vi "FGV.vi"(6 "Variant":variant, 7 "Connection Information":string, 8 "error in (no error)":errorcluster, 9 "column information":T1[](array[typedef])=[{"column name"="", "data type"=enum."Double (DBL)", "size"=0, "allow null?"=TRUE}], 10 "table":string, 11 "Enum":T3(ring)) -> (0 "error out":errorcluster, 1 "data":string[][](array[string]), 3 "tables":string[](array[string]))   [LabVIEW 2014]
uses:
  <vilib>/addons/database/NI_Database_API.lvlib
  <vilib>/addons/database/Connection.llb/Conn ObjectReference.ctl
  <vilib>/addons/database/_DB Variant To Data/Database Variant To Data.xnode
  SEQ/SeqLoop/TypeDefs/HW InOut MAP.ctl
  SEQ/SeqLoop/SeqLoop.lvlib
  SEQ/SeqLoop/Classes/STEP/STEP.lvclass
  SEQ/SeqLoop/TypeDefs/LogicParsedExpression.ctl
  SEQ/SeqLoop/TypeDefs/Sequence.ctl
  SEQ/SeqLoop/TypeDefs/Program.ctl
  <vilib>/addons/database/Connection.llb/Conn Transaction.vi
  <vilib>/addons/database/Auxilliary.llb/DB Tools Transaction.ctl
  <vilib>/addons/database/Connection.llb/DB Tools Open Connec (String).vi
  <vilib>/addons/database/Auxilliary.llb/DB Tools DataTypes.ctl
  <vilib>/addons/database/Auxilliary.llb/DB Tools Column Info.ctl
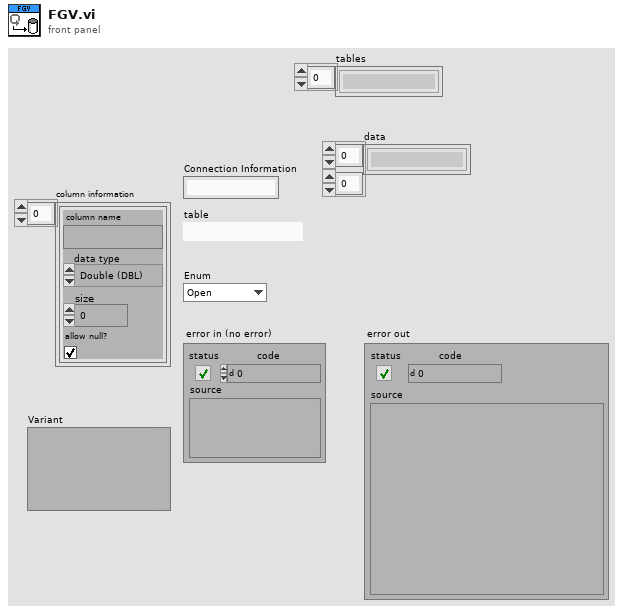
[diagram p1: front panel]
types:
  T1 = typedef "NI_Database_API.lvlib/DB Tools Column Info.ctl" = cluster{"column name":string, "data type":T2, "size":i32, "allow null?":bool}
  T2 = typedef "NI_Database_API.lvlib/DB Tools DataTypes.ctl" = enum16{"String", "Long (I32)", "Single (SGL)", "Double (DBL)", "Date/Time", "Binary"}
  T3 = enum16{"Open", "Create", "Delete", "Read_HAL", "Read_CORE", "Read_UI", "Read_MATH", "Read_SEQ", "Write_HAL", "Write_CORE", "Write_UI", "Write_MATH", "Write_SEQ", "Close"}
  T4 = typedef "NI_Database_API.lvlib/DB Tools Transaction.ctl" = enum16{"begin", "commit", "rollback"}
  T5 = typedef "NI_Database_API.lvlib/Conn ObjectReference.ctl" = refnum<k1>
  T6 = typedef "SeqLoop.lvlib/Program.ctl" = cluster{"Prog. Data":cluster{"Tipo de Programa":string, "Operación":i32, "Pieza":i32, "Descripción":string, "Nombre Programa":string, "Autor":string, "Cód. Prog.":i32, "Diseño":string, "Total Meds.:":i32, "Total Meds. Aux.:":i32}, "All Sequences":cluster{"Measurement":T7, "AutoZero":T7, "Special":T7}}
  T7 = typedef "SeqLoop.lvlib/Sequence.ctl" = cluster{"STEPs":refnum<class "STEP.lvclass">[], "Main Error&Alarm":cluster{"Main Error":T8, "Main Alarm 1":T8, "Main Alarm 2":T8, "Main Alarm 3":T8, "Main Alarm 4":T8}, "STEP Type":refnum<class "STEP.lvclass">}
  T8 = typedef "SeqLoop.lvlib/LogicParsedExpression.ctl" = cluster{"RPN ":string[], "Variables":string[], "Ctes":string[], "Formula":string, "Message":string}
  T9 = typedef "SeqLoop.lvlib/HW InOut MAP.ctl" = cluster{"Inputs":cluster{"Entrada":i32, "Descripción":string, "Habilitada?":bool}[][], "Outputs":cluster{"Salida":i32, "Descripción":string, "Habilitada?":bool, "Formula":string, "Tipo de Salida":string}[][]}
  T10 = cluster{"Entrada":i32, "Descripción":string, "Habilitada?":bool}[][]
  T11 = cluster{string, string, string, "Descripción":string, "Descripción":string}
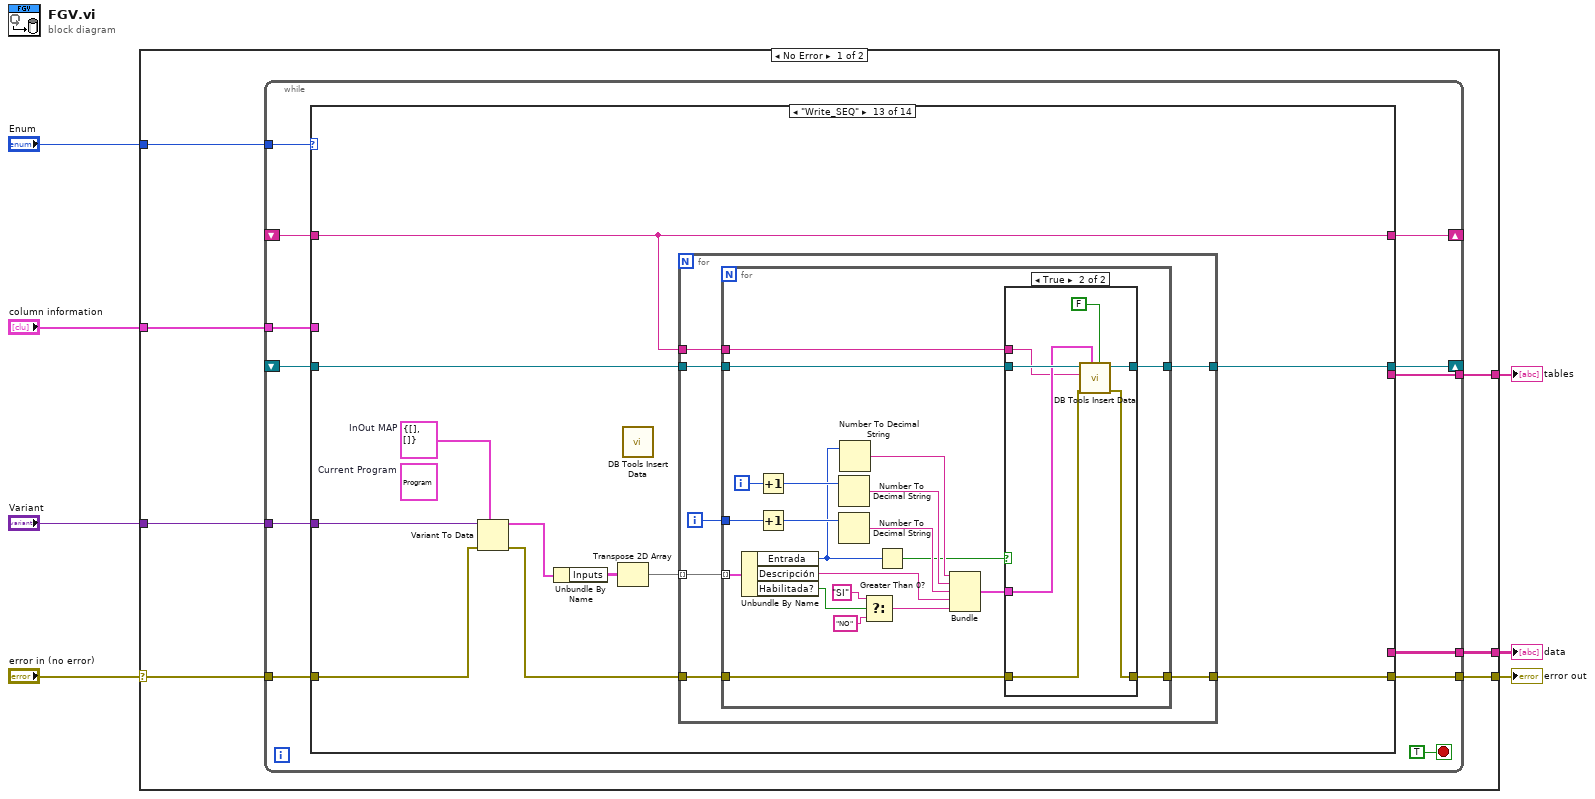
[diagram p0: block diagram]
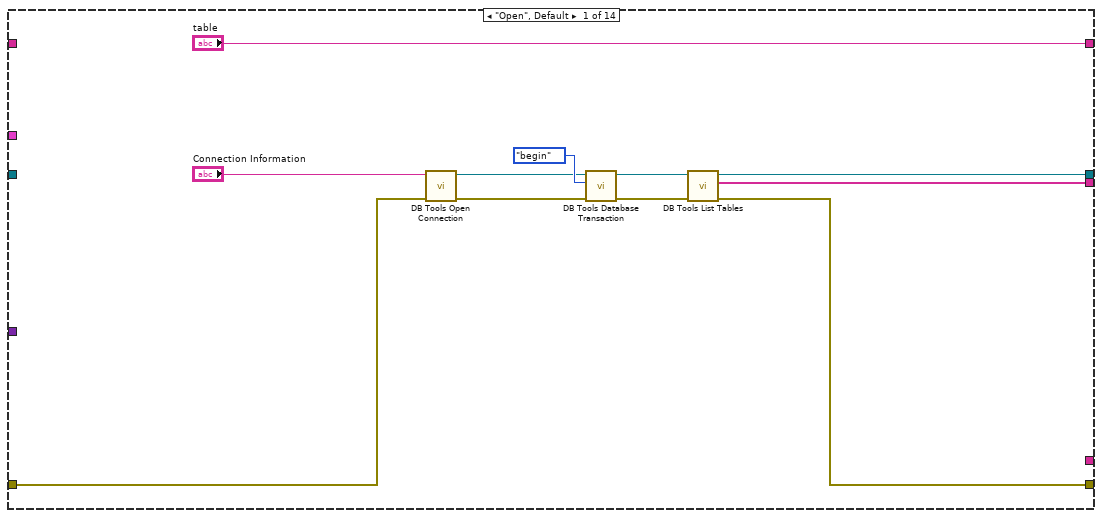
[diagram p2: hidden frame]
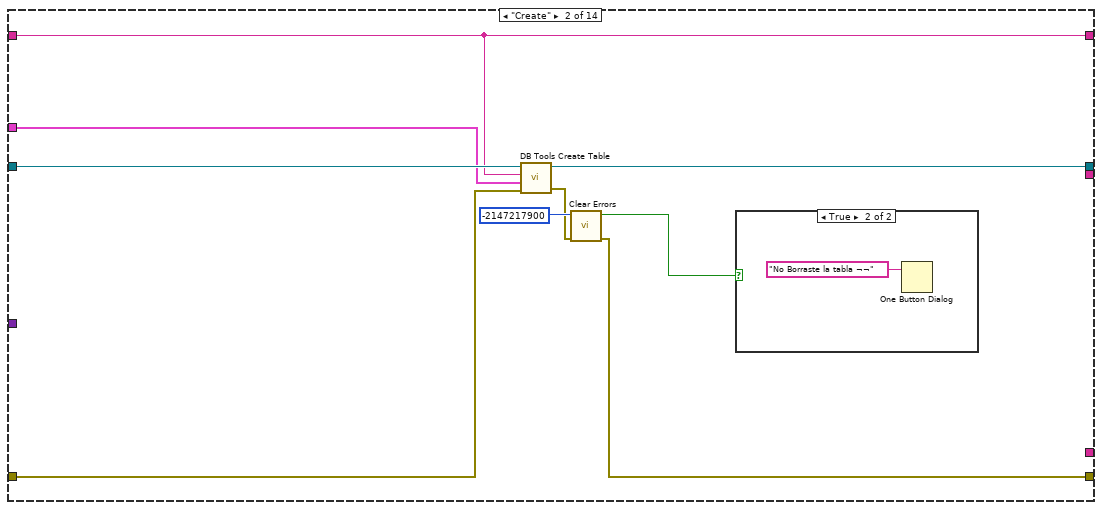
[diagram p3: hidden frame]
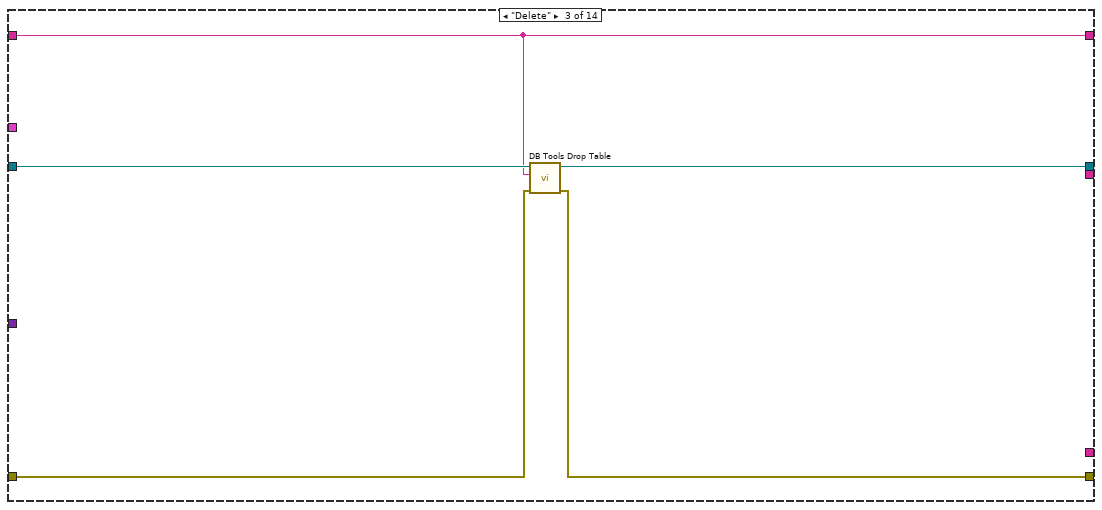
[diagram p5: hidden frame]
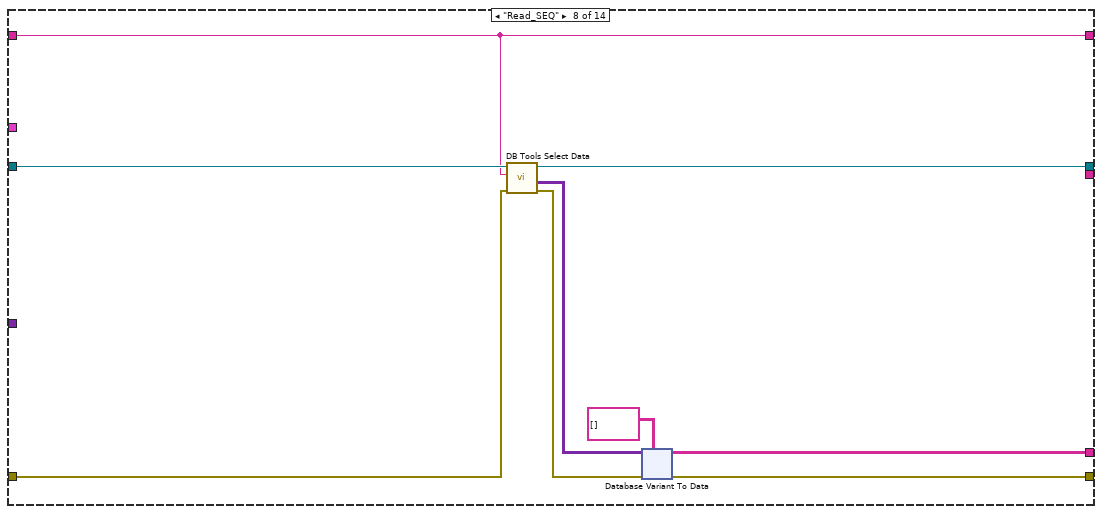
[diagram p10: hidden frame]
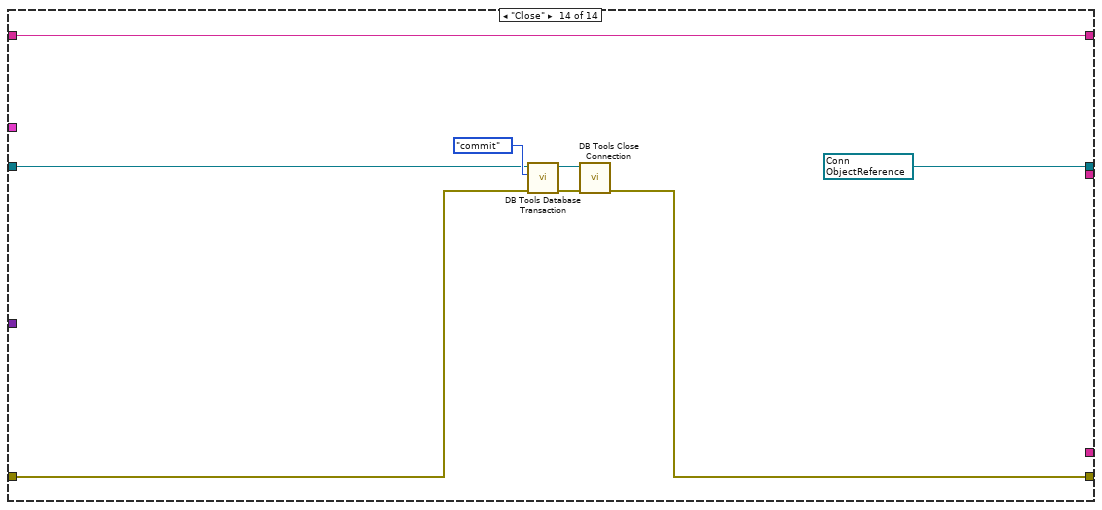
[diagram p16: hidden frame]
diagram:
  n1 = case shown="No Error" "error in (no error)" {
    selector: "error in (no error)" -> [w14 w186]
    tunnel: [w13 w186] -> w6
    tunnel: "Enum" -> [w12 _]
    tunnel: "Variant" -> [w11 _]
    tunnel: "column information" -> [w10 _]
    tunnel: [w9 _] -> w2
    tunnel: [w8 _] -> w1
    frame No Error {
      n2 = while {
        shift-right: [w24] -> _
        shift-left: _ -> [w23]
        tunnel: w12 -> [w25]
        tunnel: w14 -> [w22]
        tunnel: [w21] -> w13
        tunnel: w11 -> [w20]
        tunnel: w10 -> [w19]
        tunnel: [w17] -> w9
        shift-right: [w16] -> _
        shift-left: _ -> [w18]
        tunnel: [w15] -> w8
        stop <- TRUE stop-if-true
        n3 = case shown="\"Write_SEQ\"" w25 {
          tunnel: [w28 w44 w51 w54 w58 w61 w64 w69 w119 w123 w126 w129 w132 w184] -> w24
          tunnel: w23 -> [_ w46 w52 w54 w58 w61 w64 w70 w119 w123 w126 w129 w133 w181]
          tunnel: w22 -> [w37 w42 w49 w53 w57 w60 w63 w68 w118 w122 w125 w128 w139 w180]
          tunnel: [w30 w43 w50 w53 w57 w60 w63 w67 w118 w122 w125 w128 w131 w185] -> w21
          tunnel: w20 -> [_ _ _ _ _ _ _ _ _ _ _ _ w140 _]
          tunnel: w19 -> [_ w41 _ _ _ _ _ _ _ _ _ _ _ _]
          tunnel: w18 -> [_ w39 w48 w55 w56 w59 w62 w65 w120 w121 w124 w127 w130 w183]
          tunnel: [_ _ _ _ _ _ _ w66 _ _ _ _ _ _] -> w17
          tunnel: ["table" w39 w48 w55 w56 w59 w62 w65 w120 w121 w124 w127 w130 w183] -> w16
          tunnel: [w27 _ _ _ _ _ _ _ _ _ _ _ _ _] -> w15
          frame "Open", Default {
            n4 = call-poly <vilib>:"DB Tools Open Connection.vi"("error in (no error)"=w37, "connection information"="Connection Information") -> ("error out"=w33:errorcluster, "connection reference"=w34:T5)  [unwired: 6 in]
            n5 = call-poly <vilib>:"DB Tools Database Transaction.vi"("error in (no error)"=w33, "operation (begin)"=DB_Tools_Transaction."begin", "connection reference"=w34) -> ("error out"=w31:errorcluster, "connection reference out"=w29:T5)  [unwired: 3 in]
            n6 = call <vilib>:"DB Tools List Tables.vi"("error in (no error)"=w31, "connection reference"=w29) -> ("error out"=w30:errorcluster, "tables"=w27:string[], "connection reference out"=w28:T5)  [unwired: 3 in]
          }
          frame "Create" {
            n7 = call <vilib>:"DB Tools Create Table.vi"("error in (no error)"=w42, "column information"=w41, "table"=w39, "connection reference"=w46) -> ("error out"=w38:errorcluster, "connection reference out"=w44:T5)  [unwired: 4 in]
            n8 = call <vilib>:"Clear Errors.vi"("error in (no error)"=w38, "specific error code to clear (0: all)"=-2147217900) -> ("error out"=w43:errorcluster, "specific error cleared?"=w40:bool)  [unwired: 4 in]
            n9 = case shown="True" w40 {
              frame False {
              }
              frame True {
                n10 = One Button Dialog(message="No Borraste la tabla ¬¬") -> ()  [unwired: 1 in, 1 out]
              }
            }
          }
          frame "Delete" {
            n11 = call <vilib>:"DB Tools Drop Table.vi"("error in (no error)"=w49, "table"=w48, "connection reference"=w52) -> ("error out"=w50:errorcluster, "connection reference out"=w51:T5)  [unwired: 5 in]
          }
          frame "Read_HAL" {
          }
          frame "Read_CORE" {
          }
          frame "Read_UI" {
          }
          frame "Read_MATH" {
          }
          frame "Read_SEQ" {
            n12 = call <vilib>:"DB Tools Select Data.vi"("error in (no error)"=w68, "table"=w65, "connection reference"=w70) -> ("error out"=w71:errorcluster, "data"=w72:variant[][], "connection reference out"=w69:T5)  [unwired: 3 in]
            n13 = xnode "Database Variant To Data"("database variant"=w72, "error in (no error)"=w71, "type"=string[][] [] ("Table Control 2")) -> ("data"=w66:string[][], "error out"=w67:errorcluster)
          }
          frame "Write_HAL" {
          }
          frame "Write_CORE" {
          }
          frame "Write_UI" {
          }
          frame "Write_MATH" {
          }
          frame "Write_SEQ" {
            (unwired) T6 {"Prog. Data"={"Tipo de Programa"="", "Operación"=0, "Pieza"=0, "Descripción"="", "Nombre Programa"="", "Autor"="", "Cód. Prog."=0, "Diseño"="", "Total Meds.:"=0, "Total Meds. Aux.:"=0}, "All Sequences"={"Measurement"={"STEPs"=[], "Main Error&Alarm"={"Main Error"={"RPN "=[], "Variables"=[], "Ctes"=[], "Formula"="", "Message"=""}, "Main Alarm 1"={"RPN "=[], "Variables"=[], "Ctes"=[], "Formula"="", "Message"=""}, "Main Alarm 2"={"RPN "=[], "Variables"=[], "Ctes"=[], "Formula"="", "Message"=""}, "Main Alarm 3"={"RPN "=[], "Variables"=[], "Ctes"=[], "Formula"="", "Message"=""}, "Main Alarm 4"={"RPN "=[], "Variables"=[], "Ctes"=[], "Formula"="", "Message"=""}}, "STEP Type"=refnum}, "AutoZero"={"STEPs"=[], "Main Error&Alarm"={"Main Error"={"RPN "=[], "Variables"=[], "Ctes"=[], "Formula"="", "Message"=""}, "Main Alarm 1"={"RPN "=[], "Variables"=[], "Ctes"=[], "Formula"="", "Message"=""}, "Main Alarm 2"={"RPN "=[], "Variables"=[], "Ctes"=[], "Formula"="", "Message"=""}, "Main Alarm 3"={"RPN "=[], "Variables"=[], "Ctes"=[], "Formula"="", "Message"=""}, "Main Alarm 4"={"RPN "=[], "Variables"=[], "Ctes"=[], "Formula"="", "Message"=""}}, "STEP Type"=refnum}, "Special"={"STEPs"=[], "Main Error&Alarm"={"Main Error"={"RPN "=[], "Variables"=[], "Ctes"=[], "Formula"="", "Message"=""}, "Main Alarm 1"={"RPN "=[], "Variables"=[], "Ctes"=[], "Formula"="", "Message"=""}, "Main Alarm 2"={"RPN "=[], "Variables"=[], "Ctes"=[], "Formula"="", "Message"=""}, "Main Alarm 3"={"RPN "=[], "Variables"=[], "Ctes"=[], "Formula"="", "Message"=""}, "Main Alarm 4"={"RPN "=[], "Variables"=[], "Ctes"=[], "Formula"="", "Message"=""}}, "STEP Type"=refnum}}}  # Current Program
            w135 = T9 {"Inputs"=[], "Outputs"=[]}  # InOut MAP
            n14 = Variant To Data(error in=w139, type=w135, Variant=w140) -> (data=w134:T9, error out=w136:errorcluster)
            n15 = Unbundle By Name(w134) -> ("Inputs"=w138:T10)
            n16 = Transpose 2D Array(2D array=w138) -> (transposed array=w137:T10)
            n17 = call <vilib>:"DB Tools Insert Data.vi"() -> ()  [unwired: 10 in, 2 out]
            n18 = for {
              tunnel: w137 -> [w147] mode=indexing
              tunnel: w136 -> [w142]
              tunnel: w133 -> [w145]
              tunnel: [w144] -> w132
              tunnel: [w143] -> w131
              tunnel: w130 -> [w141]
              i -> [w146]
              n19 = for {
                tunnel: w147 -> [w168] mode=indexing
                tunnel: w146 -> [w164]
                tunnel: w145 -> [w160]
                tunnel: [w159] -> w144
                tunnel: [w158] -> w143
                tunnel: w142 -> [w157]
                tunnel: w141 -> [w150]
                i -> [w162]
                n20 = Unbundle By Name(w168) -> ("Entrada"=w149:i32, "Descripción"=w154:string, "Habilitada?"=w167:bool)
                n21 = Increment(x=w162) -> (x+1=w161:i32)
                n22 = Increment(x=w164) -> (x+1=w163:i32)
                n23 = Number To Decimal String(number=w161) -> (decimal integer string=w155:string)  [unwired: 1 in]
                n24 = Number To Decimal String(number=w163) -> (decimal integer string=w153:string)  [unwired: 1 in]
                n25 = Number To Decimal String(number=w149) -> (decimal integer string=w156:string)  [unwired: 1 in]
                n26 = Select(t="SI" ("Descripción"), s=w167, f="NO" ("Descripción")) -> (s? t:f=w152:string)
                n27 = Greater Than 0?(x=w149) -> (x > 0?=w148:bool)
                n28 = Bundle(w156, w155, w153, "Descripción"=w154, "Descripción"=w152) -> (w151:T11)  [unwired: 1 in]
                n29 = case shown="True" w148 {
                  tunnel: w160 -> [w170 w177]
                  tunnel: [w170 w176] -> w159
                  tunnel: [w169 w175] -> w158
                  tunnel: w157 -> [w169 w174]
                  tunnel: w151 -> [_ w172]
                  tunnel: w150 -> [_ w171]
                  frame False {
                  }
                  frame True {
                    n30 = call <vilib>:"DB Tools Insert Data.vi"("create table? (F)"=FALSE, "data"=w172, "error in (no error)"=w174, "table"=w171, "connection reference"=w177) -> ("error out"=w175:errorcluster, "connection reference out"=w176:T5)  [unwired: 5 in]
                  }
                }
              }
            }
          }
          frame "Close" {
            w184 = T5 refnum items=["Connection"] ("connection reference")
            n31 = call-poly <vilib>:"DB Tools Database Transaction.vi"("error in (no error)"=w180, "operation (begin)"=DB_Tools_Transaction."commit", "connection reference"=w181) -> ("error out"=w179:errorcluster, "connection reference out"=w178:T5)  [unwired: 3 in]
            n32 = call <vilib>:"DB Tools Close Connection.vi"("error in (no error)"=w179, "connection reference"=w178) -> ("error out"=w185:errorcluster)  [unwired: 5 in]
          }
        }
      }
    }
    frame Error {
    }
  }
  "error out" <- w6
  "data" <- w2
  "tables" <- w1
